vi "Packet_decode_TargetCornerArray.vi"(7 "NextByte in":i32, 9 "RawData":u8[](array[numeric])) -> (1 "NextByte out":i32, 3 "TargetCornerArray":T1[](array[typedef]))   [LabVIEW 2019, in "PhotonVisionLib.lvlib"]
doc: "Decode (or strip out) aTarget Corner Array value from the provided byte array. No conversion or decoding is actually done, the memory is just copied, and the value is cast to the correct type.\n\nInputs\n - RawData -- Array of bytes containing the data to be extracted.\n - StartByte -- The starting byte number (the first byte starts at 0)\n\nOutputs\n - Target Corner Array -- Extracted Array of Target Corner cluster.\n - NextByte -- The starting byte index for the next value (regardless of type)."
uses:
  <vilib>/Rock Robotics/WPI/ThirdParty/JAS_Junk/TrajLib/VI/Quaternion_Normalize.vi
  <vilib>/Rock Robotics/WPI/ThirdParty/JAS_Junk/TrajLib/VI/Quaternion_New_Default.vi
  PhotonVisionLib.lvlib
  TypeDef/TargetCornerType.ctl
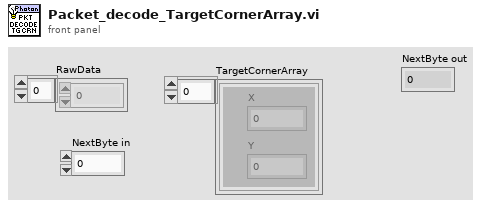
[diagram p1: front panel]
types:
  T1 = typedef "PhotonVisionLib.lvlib/TargetCornerType.ctl" = cluster{"X":dbl, "Y":dbl}
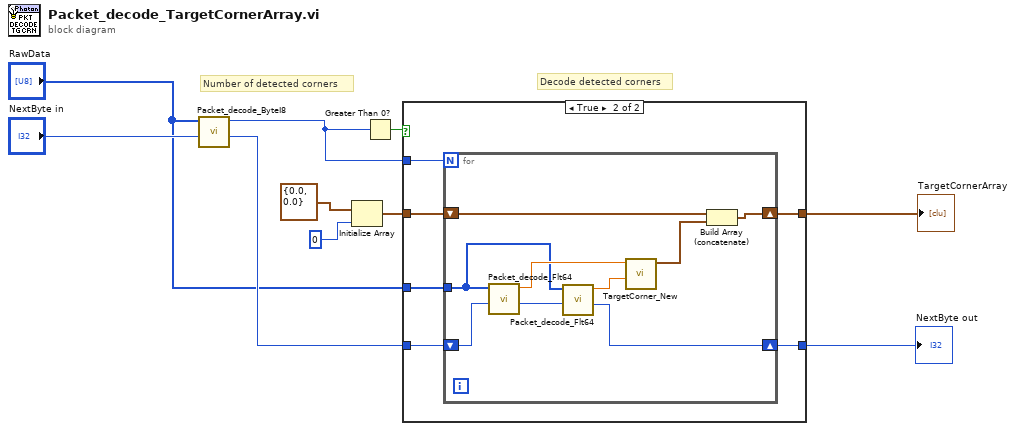
[diagram p0: block diagram]
diagram:
  # "Decode detected corners"
  # "Number of detected corners"
  n1 = call "Packet_decode_ByteI8.vi"("StartByte"="NextByte in", "RawData"="RawData") -> ("NextByte"=w6:i32, "Int8_Value"=w5:i8)  [unwired: 8 in]
  n2 = Initialize Array(T1 {"X"=0.0, "Y"=0.0} ("TargetCorner"), 0 ("dimension size")) -> (w7:T1[])
  n3 = Greater Than 0?(x=w5) -> (x > 0?=w10:bool)
  n4 = case shown="True" w10 {
    tunnel: w7 -> [w12 w17]
    tunnel: [w12 w16] -> w1
    tunnel: w6 -> [w11 w14]
    tunnel: [w11 w13] -> w2
    tunnel: w5 -> [_ w18]
    tunnel: "RawData" -> [_ w15]
    frame False {
    }
    frame True {
      n5 = for {
        N: w18 -> [_]
        shift-right: [w26] -> w16
        shift-left: w17 -> [w27]
        tunnel: w15 -> [w20]
        shift-right: [w21] -> w13
        shift-left: w14 -> [w22]
        n6 = call "Packet_decode_Flt64.vi"("StartByte"=w22, "RawData"=w20) -> ("NextByte"=w25:i32, "Flt64_Value"=w24:dbl)  [unwired: 8 in]
        n7 = call "Packet_decode_Flt64.vi"("StartByte"=w25, "RawData"=w20) -> ("NextByte"=w21:i32, "Flt64_Value"=w23:dbl)  [unwired: 8 in]
        n8 = call "TargetCorner_New.vi"("Y"=w23, "X"=w24) -> ("TargetCorner"=w19:T1)  [unwired: 9 in]
        n9 = Build Array (concatenate)(w27, w19) -> (w26:T1[])
      }
    }
  }
  "NextByte out" <- w2
  "TargetCornerArray" <- w1
